vi "AlazarErrorClusterToCode.vi"(1 "error in (no error)":errorcluster) -> (0 "Error Code":u32)   [LabVIEW 2024]
doc: "Extracts the ATS-SDK error code from a LabVIEW error cluster."
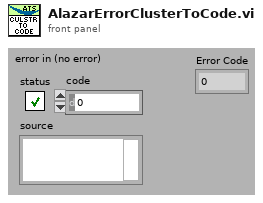
[diagram p1: front panel]
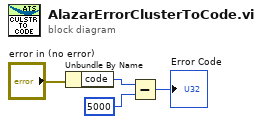
[diagram p0: block diagram]
diagram:
  n1 = Unbundle By Name("error in (no error)") -> ("code"=w3:i32)
  n2 = Subtract(x=w3, y=5000) -> (x-y=→"Error Code":i32)
